vi "Get Cell (String).vi"(8 "error in":errorcluster, 9 "Cell Address":string, 10 "Sheet Name":string, 11 "SpreadsheetDocument":refnum<k24>) -> (0 "error out":errorcluster, 2 "Value String":string, 3 "SpreadsheetDocument out":refnum<k24>)   [LabVIEW 2021, in "Open Xml.lvlib"]
uses:
  Open Xml.lvlib
  C:/Users/tupp_js/.nuget/packages/documentformat.openxml/3.3.0/lib/net46/DocumentFormat.OpenXml.dll
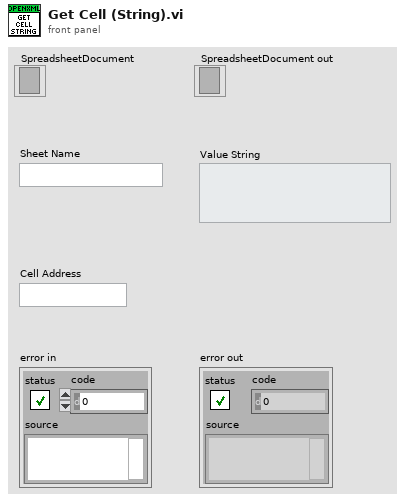
[diagram p1: front panel]
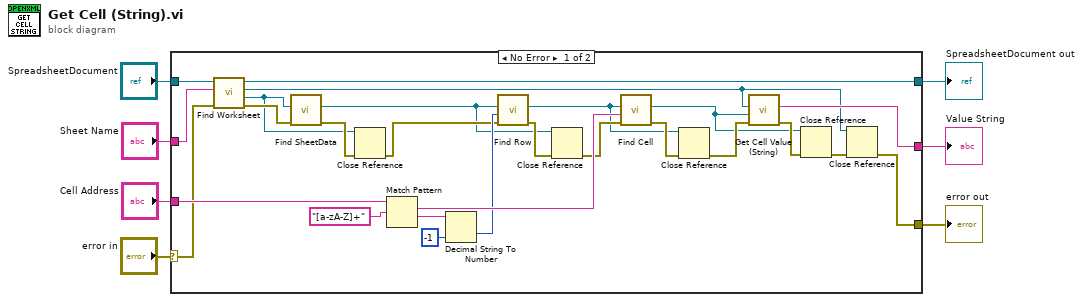
[diagram p0: block diagram]
diagram:
  n1 = case shown="No Error" "error in" {
    selector: "error in" -> [w24 w35]
    tunnel: "Sheet Name" -> [w33 _]
    tunnel: "Cell Address" -> [w31 _]
    tunnel: [w20 _] -> w4
    tunnel: [w12 w35] -> w3
    tunnel: "SpreadsheetDocument" -> [w10 w34]
    tunnel: [w8 w34] -> w1
    frame No Error {
      n2 = call "Find Worksheet.vi"("error in"=w24, "Sheet Name"=w33, "SpreadsheetDocument"=w10) -> ("error out"=w32:errorcluster, "Worksheet"=w18:refnum<k24>, "WorkbookPart"=w9:refnum<k24>, "SpreadsheetDocument out"=w8:refnum<k24>)  [unwired: 5 in]
      n3 = call "Find SheetData.vi"("error in"=w32, "Worksheet"=w18) -> ("error out"=w23:errorcluster, "SheetData"=w16:refnum<k24>)  [unwired: 8 in]
      n4 = Close Reference(reference=w18, error in (no error)=w23) -> (error out=w19:errorcluster)
      n5 = Match Pattern(string=w31, regular expression="[a-zA-Z]+") -> (match substring=w29:string, after substring=w28:string)  [unwired: 1 in, 2 out]
      n6 = Decimal String To Number(string=w28, default (0L)=-1 ("default (0 I32)")) -> (number=w27:i32)  [unwired: 1 in, 1 out]
      n7 = call "Find Row.vi"("error in"=w19, "Index"=w27, "SheetData"=w16) -> ("error out"=w21:errorcluster, "Row"=w14:refnum<k24>)  [unwired: 7 in]
      n8 = Close Reference(reference=w16, error in (no error)=w21) -> (error out=w17:errorcluster)
      n9 = call "Find Cell.vi"("error in"=w17, "Lexical Index"=w29, "Row"=w14) -> ("error out"=w22:errorcluster, "Cell"=w11:refnum<k24>)  [unwired: 7 in]
      n10 = Close Reference(reference=w14, error in (no error)=w22) -> (error out=w15:errorcluster)
      n11 = call "Get Cell Value (String).vi"("error in"=w15, "Cell"=w11, "Workbookpart"=w9) -> ("error out"=w25:errorcluster, "Value String"=w20:string)  [unwired: 7 in]
      n12 = Close Reference(reference=w11, error in (no error)=w25) -> (error out=w13:errorcluster)
      n13 = Close Reference(reference=w9, error in (no error)=w13) -> (error out=w12:errorcluster)
    }
    frame Error {
    }
  }
  "error out" <- w3
  "Value String" <- w4
  "SpreadsheetDocument out" <- w1
